vi "2 Don't Flip Setpoints.vi"(11 "Robot Pitch/Roll\nfrom Global":T1 {"Roll" format="%05.1f"; "Pitch" format="%05.1f"}) -> (2 "Tipping?":bool, 3 "Setpoint Cluster":T2)   [LabVIEW 2011]
doc: "This VI simply outputs constant sail and rudder setpoints with priority set by the input. These setpoints will be used if no other higher priority think function outputs true priority.\nThis VI takes over control as soon as the boat is over an angle of 45/ -45 degrees.\nDepending on the wind direction, the sail will be taken out of the wind, causing the boat to flip back.\n[During that time, the Rudder is locked to 0 deg, to avoid turning further into the wind.]-not anymore - we think this function was doing more harm than good.\nwritten by: Olli"
uses:
  2 Typedefs/setpoints to arbiter.ctl
  2 Typedefs/pitch and roll.ctl
  2 Typedefs/apparent wind direction.ctl
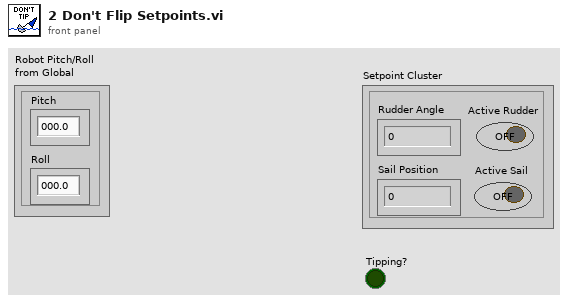
[diagram p1: front panel]
types:
  T1 = typedef "pitch and roll.ctl" = cluster{"Pitch":dbl, "Roll":dbl}
  T2 = typedef "setpoints to arbiter.ctl" = cluster{"Rudder Angle":dbl, "Sail Position":dbl, "Active Rudder":bool, "Active Sail":bool}
  T3 = typedef "apparent wind direction.ctl" = dbl
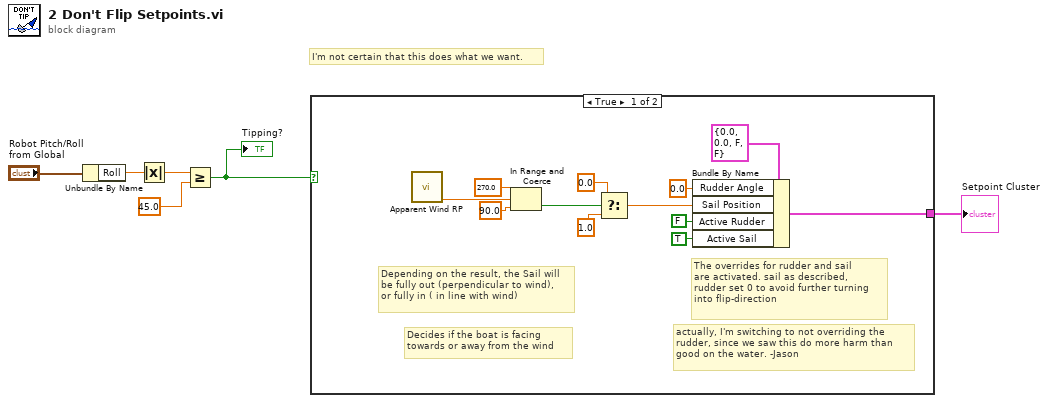
[diagram p0: block diagram]
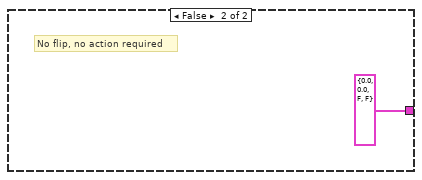
[diagram p2: hidden frame]
diagram:
  # "I'm not certain that this does what we want."
  n1 = Unbundle By Name("Robot Pitch/Roll\nfrom Global") -> ("Roll"=w4:dbl)
  n2 = Absolute Value(x=w4) -> (abs(x)=w3:dbl)
  n3 = Greater Or Equal?(x=w3, y=45.0) -> (x >= y?=w1:bool)
  "Tipping?" <- w1
  n4 = case shown="True" w1 {
    tunnel: [w13 T2 {"Rudder Angle"=0.0, "Sail Position"=0.0, "Active Rudder"=FALSE, "Active Sail"=FALSE} ("Setpoint Cluster")] -> w6
    frame True {
      # "actually, I'm switching to not overriding the\nrudder, since we saw this do more harm than\ngood on the water. -Jason"
      # "The overrides for rudder and sail \nare activated. sail as described,\nrudder set 0 to avoid further turning \ninto flip-direction"
      # "Depending on the result, the Sail will\nbe fully out (perpendicular to wind),\nor fully in ( in line with wind)"
      # "Decides if the boat is facing \ntowards or away from the wind"
      n5 = call "Apparent Wind RP.vi"() -> ("Apparent Wind Direction RP"=w7:dbl)  [unwired: 8 in, 3 out]
      n6 = In Range and Coerce(upper limit=T3 270.0, x=w7, lower limit=T3 90.0) -> (In Range?=w9:bool)  [unwired: 1 out]
      n7 = Select(t=0.0, s=w9, f=1.0) -> (s? t:f=w14:dbl)
      n8 = Bundle By Name(cluster=T2 {"Rudder Angle"=0.0, "Sail Position"=0.0, "Active Rudder"=FALSE, "Active Sail"=FALSE} ("Setpoint Cluster"), "Rudder Angle"=0.0, "Sail Position"=w14, "Active Rudder"=FALSE, "Active Sail"=TRUE ("Use Defaults")) -> (w13:T2)
    }
    frame False {
      # "No flip, no action required"
    }
  }
  "Setpoint Cluster" <- w6
